vi "Read Value.vi"(8 "error in (no error)":errorcluster, 11 "int32 in":refnum<class "uint32.lvclass">) -> (0 "error out":errorcluster, 2 "Value":u32, 3 "int32 out":refnum<class "uint32.lvclass">)   [LabVIEW 2020, in "Protobuf RAW.lvlib" / "uint32.lvclass"]
uses:
  uint32.lvclass
  uint32.lvclass/uint32.ctl
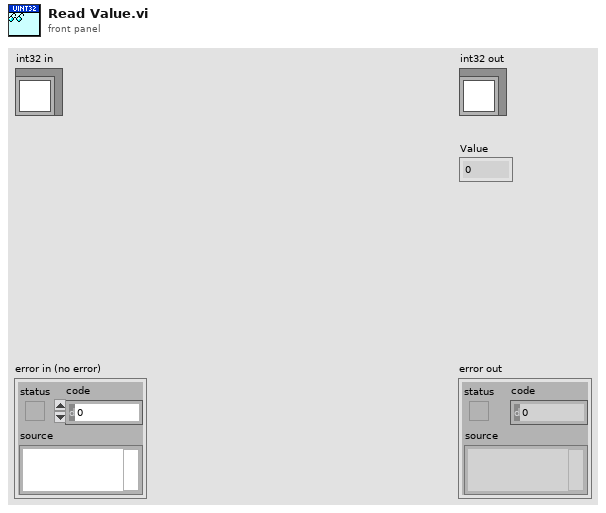
[diagram p1: front panel]
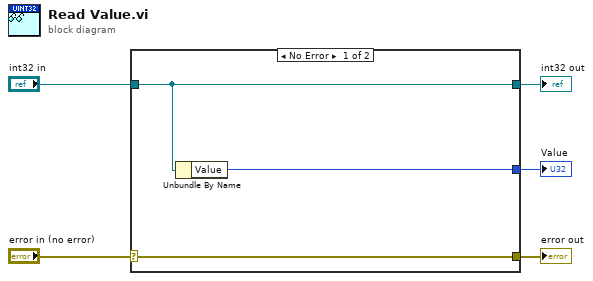
[diagram p0: block diagram]
diagram:
  n1 = case shown="No Error" "error in (no error)" {
    selector: "error in (no error)" -> [w8 w9]
    tunnel: [w8 w9] -> w4
    tunnel: [w7 w10] -> w2
    tunnel: "int32 in" -> [w7 w10]
    tunnel: [w6 _] -> w1
    frame No Error {
      n2 = Unbundle By Name(w7) -> ("Value"=w6:u32)
    }
    frame Error {
    }
  }
  "error out" <- w4
  "int32 out" <- w2
  "Value" <- w1
